vi "modbus验证_控制可调电源.vi"() -> ()   [LabVIEW 2020]
uses:
  <vilib>/Plasmionique/MB Master/MB_Master_Serial/MB_Master_Serial.lvclass
  C:/Program Files (x86)/National Instruments/LabVIEW 2020/vi.lib/Plasmionique/MB Master/MB_Master/MB_Master.lvclass
  <vilib>/Plasmionique/MB Master/MB Master.lvlib
panel:
  in  "停止":bool
  out "目标输出电压":dbl format="%#_5f V"
  in  "转盘":i16(knob) scale=100.0..1400.0
  out "error out":errorcluster
  out "仪表":dbl(knob) scale=100.0..1400.0
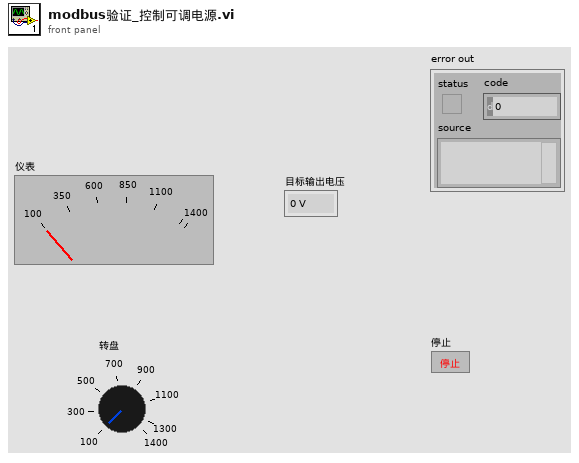
[diagram p1: front panel]
types:
  T1 = cluster{"baud rate (bps)":u32, "stop bits":u16, "parity":u16, "flow control":u16, "timeout":u32, "retries":i32}
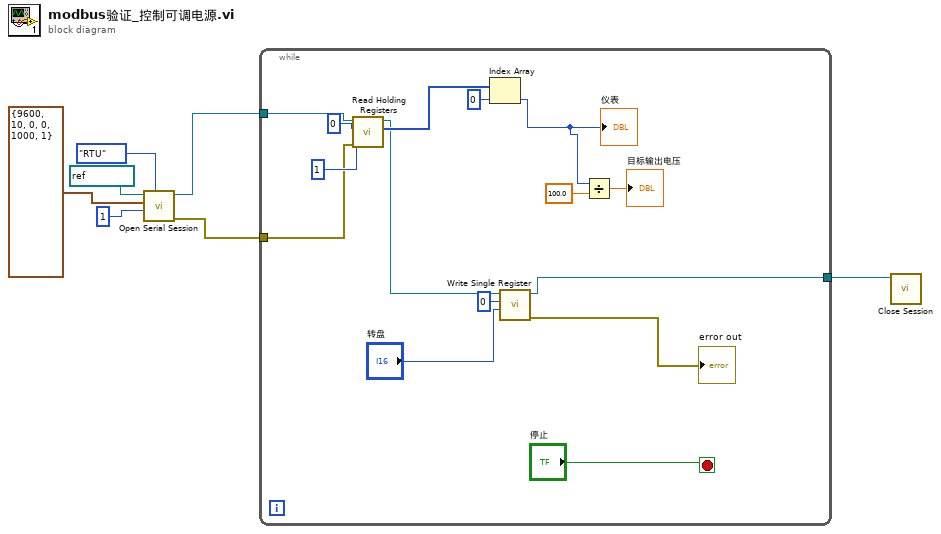
[diagram p0: block diagram]
diagram:
  n1 = call <vilib>:"Open Serial Session.vi"("Mode (RTU)"=enum16{"RTU", "ASCII"}."RTU", "Slave ID"=u8 1, "Serial Config"=T1 {"baud rate (bps)"=9600, "stop bits"=10, "parity"=0, "flow control"=0, "timeout"=1000, "retries"=1}, "VISA Resource"=refnum<visa-resource-name> "COM4") -> ("Error out"=w2:errorcluster, "MB_Serial session"=w3:refnum<class "MB_Master_Serial.lvclass">)  [unwired: 6 in]
  n2 = while {
    tunnel: w3 -> [w22]
    tunnel: w2 -> [w19]
    tunnel: [w9] -> w1
    stop <- "停止" stop-if-true
    n3 = call <vilib>:"Read Holding Registers.vi"("error in (no error)"=w19, "quantity"=u16 1, "starting address"=u16 0, "MB session in"=w22) -> ("Registers"=w18:u16[], "MB session out"=w16:refnum<class "MB_Master_Serial.lvclass">)  [unwired: 5 in, 1 out]
    n4 = Index Array(array=w18, index=0 ("索引")) -> (element=w11:u16)
    "仪表" <- w11
    n5 = call <vilib>:"Write Single Register.vi"("value"="转盘", "address"=u16 0, "MB session in"=w16) -> ("error out"=→"error out":errorcluster, "MB session out"=w9:refnum<class "MB_Master_Serial.lvclass">)  [unwired: 7 in]
    n6 = Divide(x=w11, y=100.0) -> (x/y=→"目标输出电压":dbl)
  }
  n7 = call-dynamic "Close Session.vi"("MB_Serial session"=w1) -> ()  [unwired: 10 in, 1 out]
